vi "RandomBoolArray.vi"(1 "random array size":i32=256) -> (0 "random array":bool[](array[boolean]))   [LabVIEW 2009]
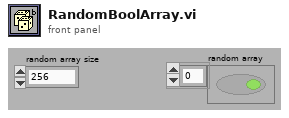
[diagram p1: front panel]
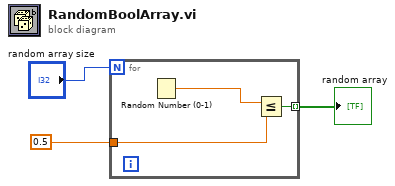
[diagram p0: block diagram]
diagram:
  n1 = for {
    N: "random array size" -> [_]
    tunnel: 0.5 ("y") -> [w5]
    tunnel: [w4] -> w1 mode=indexing
    n2 = Random Number (0-1)() -> (number: 0 to 1=w6:dbl)
    n3 = Less Or Equal?(x=w6, y=w5) -> (x <= y?=w4:bool)
  }
  "random array" <- w1
